vi "check_hbridge.vi"(6 "timeout (25000ms)":i32=25000, 8 "error in (no error)":errorcluster, 11 "daemon reference in":refnum<k5>) -> (0 "error out":errorcluster, 2 "response":string, 3 "daemon reference out":refnum<k5>, 5 "command out":string="random")   [LabVIEW 2017]
doc: "<b>Command: </b>\"check_hbridge\"\n\n<b>Description: </b> This command will perform a bridge check\n\n<b>Parameters: </b> None\n____________________________________________\nDIPC 692 Daemon API 10.0.0.1\nSam Tee - Dyson Technology Ltd\nCopyright (c) 2024, Dyson Technology Ltd"
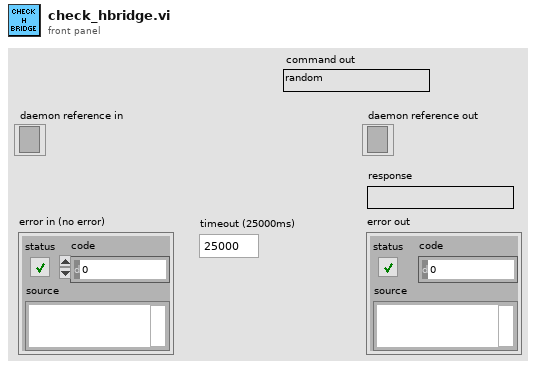
[diagram p1: front panel]
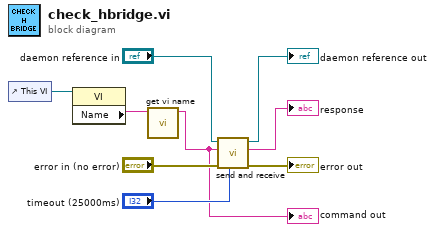
[diagram p0: block diagram]
diagram:
  n1 = control-ref of="This VI"() -> (w3:refnum<vi>)
  n2 = property class="VI"(reference=w3) -> ("Name"=w2:string)  [unwired: 1 in, 2 out]
  n3 = call "get vi name.vi"("library.lvlib:name.vi"=w2) -> ("vi name"=w1:string)  [unwired: 10 in]
  "command out" <- w1
  n4 = call "send and receive.vi"("timeout (25000ms)"="timeout (25000ms)", "error in (no error)"="error in (no error)", "command"=w1, "daemon reference in"="daemon reference in") -> ("error out"=→"error out":errorcluster, "response"=→"response":string, "daemon reference out"=→"daemon reference out":refnum<k5>)  [unwired: 5 in]
